vi "HEWH Tank Display.vi"(0 "Local Tank Display":refnum<vi>, 5 "T1-T6.Tin,Tout":dbl[](array[numeric]), 7 "Min Temp (°F)":dbl=50.0, 9 "Max Temp (°F)":dbl=140.0, 11 "error in":errorcluster) -> (15 "error out":errorcluster)   [LabVIEW 2012]
uses:
  HEWH Tank Indicator.ctl
  <vilib>/Analysis/NI_AALBase.lvlib
panel:
  in  "Tank Display":T1 {"TC6" format="%.2g"; "TIN" format="%.2g"; "TOUT" format="%.2g"; "Mean" format="%.2f"; "Std Dev" format="%.2f"; "TC5" format="%.2g"; "TC4" format="%.2g"; "TC3" format="%.2g"; "TC2" format="%.2g"; "TC1" format="%.2g"}
  out "Array 2":string[](array[string])
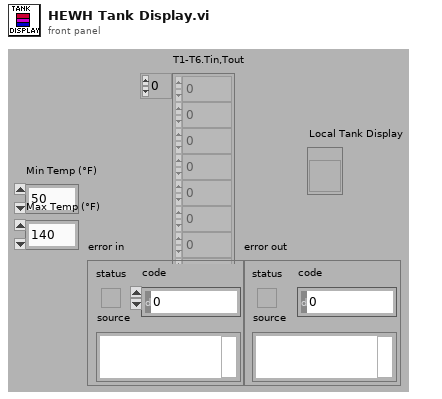
[diagram p1: front panel]
types:
  T1 = typedef "HEWH Tank Indicator.ctl" = cluster{"TC1-D":bool, "TC2-D":bool, "TC3-D":bool, "TC4-D":bool, "TC5-D":bool, "RTD_IN":bool, "RTDOUT":bool, "TC1":dbl, "TC2":dbl, "TC3":dbl, "TC4":dbl, "TC5":dbl, "TIN":dbl, "TOUT":dbl, "Std Dev":dbl, "Mean":dbl, "TC6-D":bool, "TC6":dbl}
  T2 = cluster{"T1-T6.Tin,Tout[0]":dbl, "T1-T6.Tin,Tout[1]":dbl, "T1-T6.Tin,Tout[2]":dbl, "T1-T6.Tin,Tout[3]":dbl, "T1-T6.Tin,Tout[4]":dbl, "T1-T6.Tin,Tout[5]":dbl, "T1-T6.Tin,Tout[6]":dbl, "T1-T6.Tin,Tout[7]":dbl}
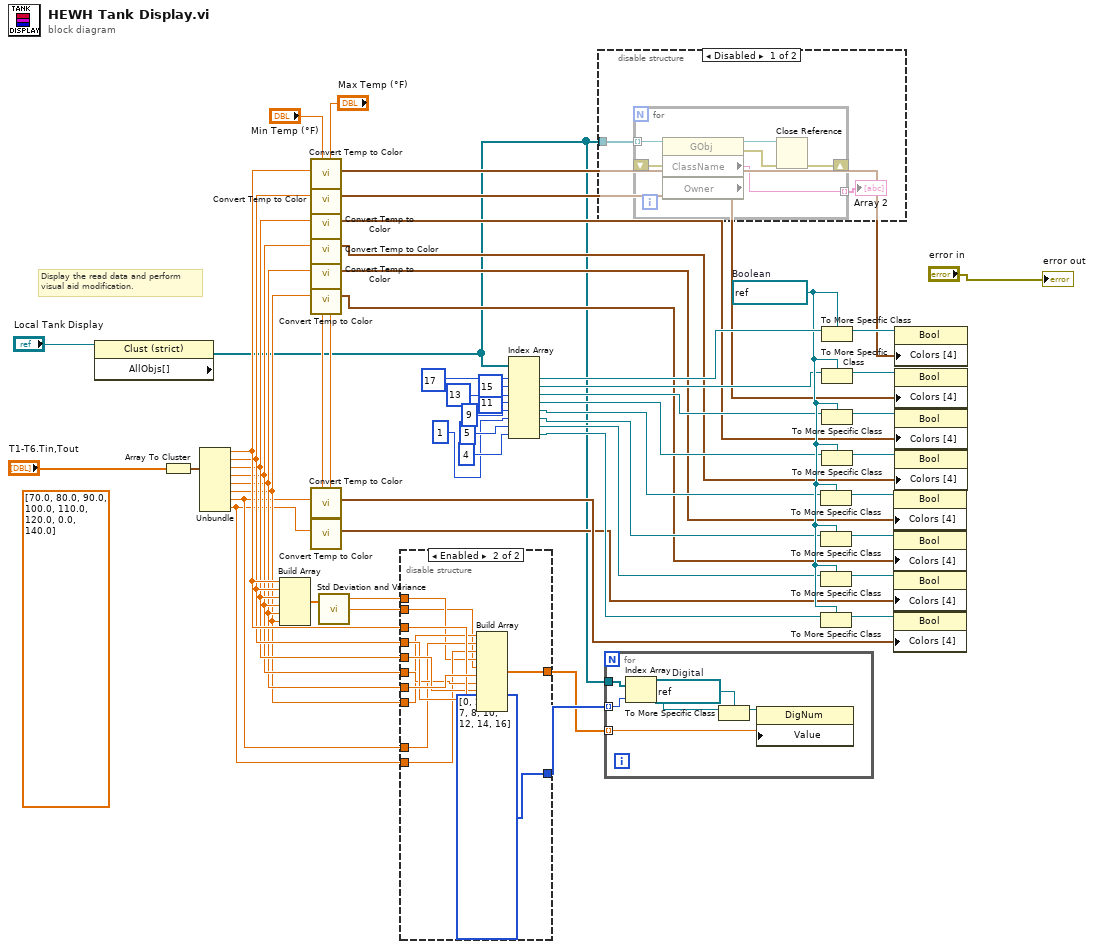
[diagram p0: block diagram]
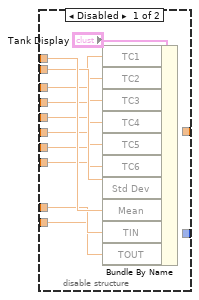
[diagram p2: hidden frame]
diagram:
  (unwired) dbl[] [70.0, 80.0, 90.0, 100.0, 110.0, 120.0, 0.0, 140.0] ("array")
  w31 = refnum<vi> refnum  # Boolean
  # "Display the read data and perform\nvisual aid modification."
  n1 = property class="Clust (strict)"(reference="Local Tank Display") -> ("AllObjs[]"=w6:refnum<vi>[])  [unwired: 1 in, 2 out]
  n2 = Array To Cluster(array="T1-T6.Tin,Tout") -> (cluster=w57:T2)
  n3 = Unbundle(w57) -> ("T1-T6.Tin,Tout[0]"=w44:dbl, "T1-T6.Tin,Tout[1]"=w43:dbl, "T1-T6.Tin,Tout[2]"=w42:dbl, "T1-T6.Tin,Tout[3]"=w41:dbl, "T1-T6.Tin,Tout[4]"=w40:dbl, "T1-T6.Tin,Tout[5]"=w39:dbl, "T1-T6.Tin,Tout[6]"=w12:dbl, "T1-T6.Tin,Tout[7]"=w11:dbl)
  n4 = Build Array(w44, w43, w42, w41, w40, w39) -> (w7:dbl[])
  n5 = call "Convert Temp to Color.vi"("Max Temp (°F)"="Max Temp (°F)", "Min Temp (°F)"="Min Temp (°F)", "Temp (°F)"=w44) -> ("Color Output"=w51:cluster{"Color":u32, "Color":u32}[], "Max Temp (°F) Out"=w59:dbl, "Min Temp (°F) Out"=w58:dbl)  [unwired: 6 out]
  n6 = call "Convert Temp to Color.vi"("Max Temp (°F)"=w59, "Min Temp (°F)"=w58, "Temp (°F)"=w43) -> ("Color Output"=w23:cluster{"Color":u32, "Color":u32}[], "Max Temp (°F) Out"=w61:dbl, "Min Temp (°F) Out"=w60:dbl)  [unwired: 6 out]
  n7 = call "Convert Temp to Color.vi"("Max Temp (°F)"=w61, "Min Temp (°F)"=w60, "Temp (°F)"=w42) -> ("Color Output"=w22:cluster{"Color":u32, "Color":u32}[], "Max Temp (°F) Out"=w63:dbl, "Min Temp (°F) Out"=w62:dbl)  [unwired: 6 out]
  n8 = call "Convert Temp to Color.vi"("Max Temp (°F)"=w63, "Min Temp (°F)"=w62, "Temp (°F)"=w41) -> ("Color Output"=w21:cluster{"Color":u32, "Color":u32}[], "Max Temp (°F) Out"=w65:dbl, "Min Temp (°F) Out"=w64:dbl)  [unwired: 6 out]
  n9 = call "Convert Temp to Color.vi"("Max Temp (°F)"=w65, "Min Temp (°F)"=w64, "Temp (°F)"=w40) -> ("Color Output"=w20:cluster{"Color":u32, "Color":u32}[], "Max Temp (°F) Out"=w67:dbl, "Min Temp (°F) Out"=w66:dbl)  [unwired: 6 out]
  n10 = call "Convert Temp to Color.vi"("Max Temp (°F)"=w67, "Min Temp (°F)"=w66, "Temp (°F)"=w39) -> ("Color Output"=w19:cluster{"Color":u32, "Color":u32}[], "Max Temp (°F) Out"=w17:dbl, "Min Temp (°F) Out"=w18:dbl)  [unwired: 6 out]
  n11 = call "Convert Temp to Color.vi"("Max Temp (°F)"=w17, "Min Temp (°F)"=w18, "Temp (°F)"=w12) -> ("Color Output"=w10:cluster{"Color":u32, "Color":u32}[], "Max Temp (°F) Out"=w15:dbl, "Min Temp (°F) Out"=w16:dbl)  [unwired: 6 out]
  n12 = call "Convert Temp to Color.vi"("Max Temp (°F)"=w15, "Min Temp (°F)"=w16, "Temp (°F)"=w11) -> ("Color Output"=w9:cluster{"Color":u32, "Color":u32}[])  [unwired: 8 out]
  n13 = call <vilib>:"Std Deviation and Variance.vi"("X"=w7) -> ("mean"=w56:dbl, "standard deviation"=w55:dbl)  [unwired: 1 in, 1 out]
  n14 = disable-structure shown="Enabled" {
    disable-tunnel: w56 -> [w78 w80]
    disable-tunnel: w55 -> [w77 w79]
    disable-tunnel: w44 -> [w76 w87]
    disable-tunnel: w43 -> [w75 w85]
    disable-tunnel: w42 -> [w74 w86]
    disable-tunnel: w41 -> [w73 w84]
    disable-tunnel: w40 -> [w72 w90]
    disable-tunnel: w39 -> [w71 w83]
    disable-tunnel: w12 -> [w70 w82]
    disable-tunnel: w11 -> [w69 w81]
    disable-tunnel: [_ i32[] [0, 2, 3, 6, 7, 8, 10, 12, 14, 16] ("Array")] -> w5
    disable-tunnel: [_ w88] -> w4
    frame Disabled {
      n15 = Bundle By Name(cluster="Tank Display", "TC1"=w76, "TC2"=w75, "TC3"=w74, "TC4"=w73, "TC5"=w72, "TC6"=w71, "Std Dev"=w77, "Mean"=w78, "TIN"=w70, "TOUT"=w69) -> ()  [unwired: 1 out]
    }
    frame Enabled {
      n16 = Build Array(w83, w82, w81, w80, w79, w90, w84, w86, w85, w87) -> (w88:dbl[])
    }
  }
  n17 = Index Array(array=w6, index #1=17 ("index"), index #2=15 ("index"), index #3=13 ("index"), index #4=11 ("index"), index #5=9 ("index"), index #6=1 ("index"), index #7=5 ("index"), index #8=4 ("index")) -> (element #1=w53:refnum<vi>, element #2=w30:refnum<vi>, element #3=w29:refnum<vi>, element #4=w28:refnum<vi>, element #5=w27:refnum<vi>, element #6=w26:refnum<vi>, element #7=w25:refnum<vi>, element #8=w24:refnum<vi>)
  n18 = disable-structure shown="Disabled" {
    disable-tunnel: w6 -> [w91 _]
    frame Disabled {
      n19 = for {
        tunnel: w91 -> [w95] mode=indexing
        shift-right: [w98] -> _
        shift-left: _ -> [w94]
        tunnel: [w97] -> w92 mode=indexing
        n20 = property on="Property Node" class="GObj" props=["ClassName", "Owner"](reference=w95, error in=w94) -> (reference out=w93:refnum<vi>, error out=w96:errorcluster, "ClassName"=w97:string)  [unwired: 1 out]
        n21 = Close Reference(reference=w93, error in (no error)=w96) -> (error out=w98:errorcluster)
      }
      "Array 2" <- w92
    }
    frame Enabled {
      # "This is used to find bools in cluster.  Note\nbug in Labview doesnt show array cluster\nobjects in correct order."
    }
  }
  n22 = for {
    tunnel: w6 -> [w103]
    tunnel: w5 -> [w100] mode=indexing
    tunnel: w4 -> [w99] mode=indexing
    w104 = refnum<vi> refnum  # Digital
    n23 = Index Array(array=w103, index=w100) -> (element=w102:refnum<vi>)
    n24 = To More Specific Class(target class=w104, reference=w102) -> (specific class reference=w101:refnum<vi>)  [unwired: 1 in, 1 out]
    n25 = property on="Property Node" class="DigNum"(reference=w101, "Value"=w99) -> ()  [unwired: 1 in, 2 out]
  }
  n26 = To More Specific Class(target class=w31, reference=w27) -> (specific class reference=w35:refnum<vi>)  [unwired: 1 in, 1 out]
  n27 = To More Specific Class(target class=w31, reference=w26) -> (specific class reference=w34:refnum<vi>)  [unwired: 1 in, 1 out]
  n28 = To More Specific Class(target class=w31, reference=w25) -> (specific class reference=w33:refnum<vi>)  [unwired: 1 in, 1 out]
  n29 = To More Specific Class(target class=w31, reference=w24) -> (specific class reference=w32:refnum<vi>)  [unwired: 1 in, 1 out]
  n30 = To More Specific Class(target class=w31, reference=w53) -> (specific class reference=w52:refnum<vi>)  [unwired: 1 in, 1 out]
  n31 = To More Specific Class(target class=w31, reference=w30) -> (specific class reference=w38:refnum<vi>)  [unwired: 1 in, 1 out]
  n32 = To More Specific Class(target class=w31, reference=w29) -> (specific class reference=w37:refnum<vi>)  [unwired: 1 in, 1 out]
  n33 = To More Specific Class(target class=w31, reference=w28) -> (specific class reference=w36:refnum<vi>)  [unwired: 1 in, 1 out]
  n34 = property on="Property Node" class="Bool"(reference=w35, "Colors [4]"=w20) -> ()  [unwired: 1 in, 2 out]
  n35 = property on="Property Node" class="Bool"(reference=w34, "Colors [4]"=w19) -> ()  [unwired: 1 in, 2 out]
  n36 = property on="Property Node" class="Bool"(reference=w33, "Colors [4]"=w9) -> ()  [unwired: 1 in, 2 out]
  n37 = property on="Property Node" class="Bool"(reference=w32, "Colors [4]"=w10) -> ()  [unwired: 1 in, 2 out]
  n38 = property on="Property Node" class="Bool"(reference=w52, "Colors [4]"=w51) -> ()  [unwired: 1 in, 2 out]
  n39 = property on="Property Node" class="Bool"(reference=w38, "Colors [4]"=w23) -> ()  [unwired: 1 in, 2 out]
  n40 = property on="Property Node" class="Bool"(reference=w37, "Colors [4]"=w22) -> ()  [unwired: 1 in, 2 out]
  n41 = property on="Property Node" class="Bool"(reference=w36, "Colors [4]"=w21) -> ()  [unwired: 1 in, 2 out]
  "error out" <- "error in"
